vi "include_liblinear.vi"   [LabVIEW 2014]
uses:
  bin/x64/liblinear.dll
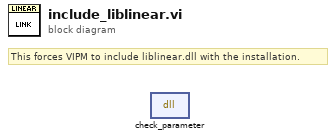
[diagram p0: block diagram]
diagram:
  # "This forces VIPM to include liblinear.dll with the installation."
  n1 = dll-call lib="C:/dev/LVLibSVM/LabVIEW/bin/x64/liblinear.dll" fn="check_parameter"() -> ()  [unwired: 4 in, 2 out]
